vi "Example_RCM.vi"() -> ()   [LabVIEW 2009]
uses:
  RCM.xctl
panel:
  out "Selected?":bool
  in  "Get":bool
  out "Selected Item":string caption="Selected Item:"
  in  "Stop":bool
  in  "Overlay Color":u32(colorbox)=26367 caption="Overlay Color:"
  in  "Frame Color":u32(colorbox)=9868950 caption="Frame Color:"
  in  "Seperator Color":u32(colorbox)=9868950 caption="Separator Color:"
  in  "Font Color":u32(colorbox) caption="Font Color:"
  in  "Font Size":i16=13 caption="Font Size:"
  in  "Font Name":string="Tahoma" caption="Font Name:"
  in  "RCM File Path":path caption="RCM File Path:"
  in  "Control with RCM":bool
  in  "RCM":string(xcontrol)
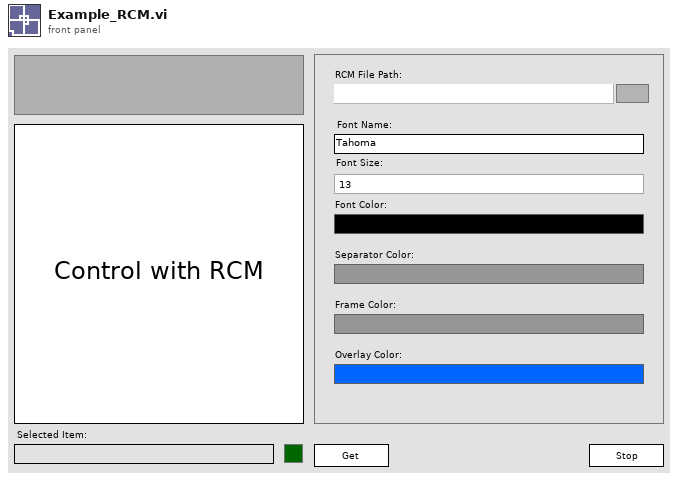
[diagram p1: front panel]
types:
  T1 = typedef "LVPoint32TypeDef.ctl" = cluster{"Horizontal":i32, "Vertical":i32}
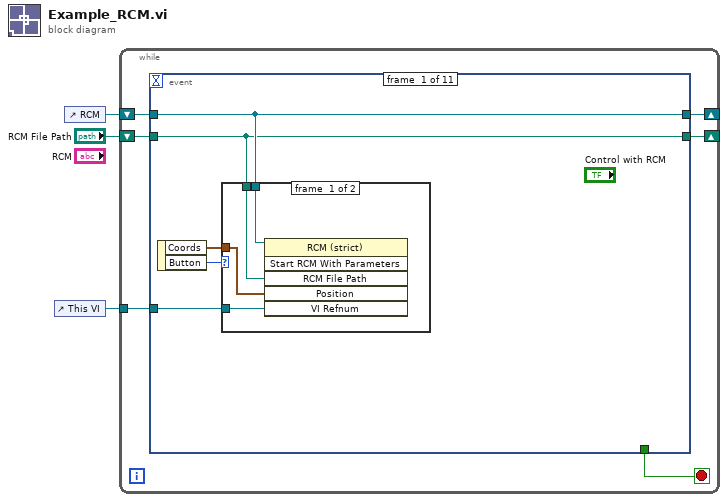
[diagram p0: block diagram]
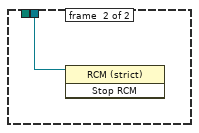
[diagram p2: hidden frame]
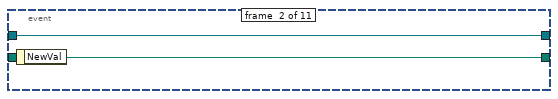
[diagram p3: hidden frame]
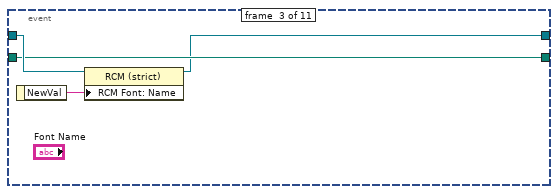
[diagram p4: hidden frame]
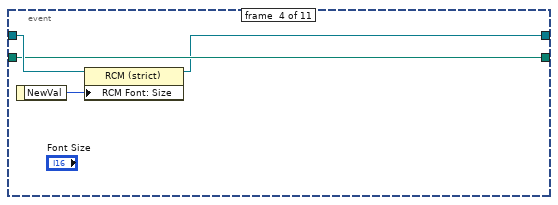
[diagram p5: hidden frame]
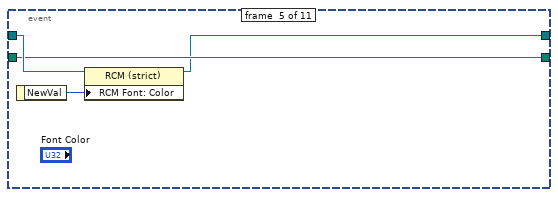
[diagram p6: hidden frame]
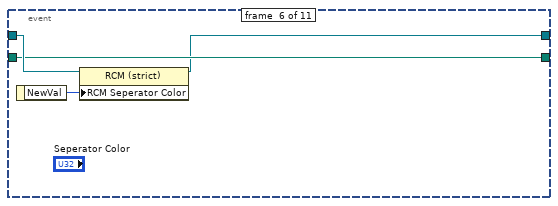
[diagram p7: hidden frame]
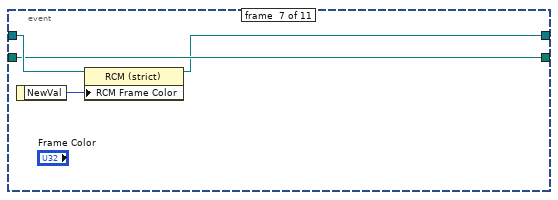
[diagram p8: hidden frame]
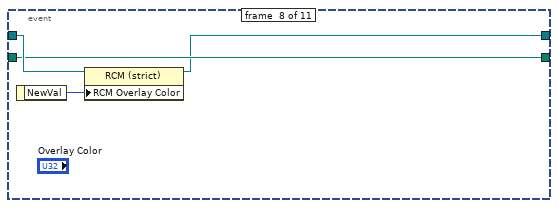
[diagram p9: hidden frame]
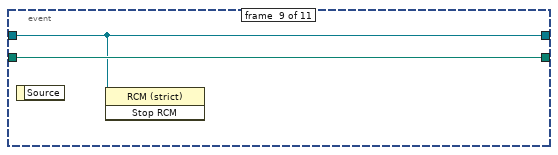
[diagram p10: hidden frame]
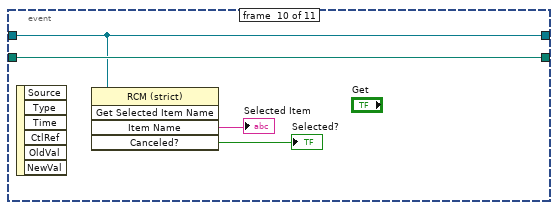
[diagram p11: hidden frame]
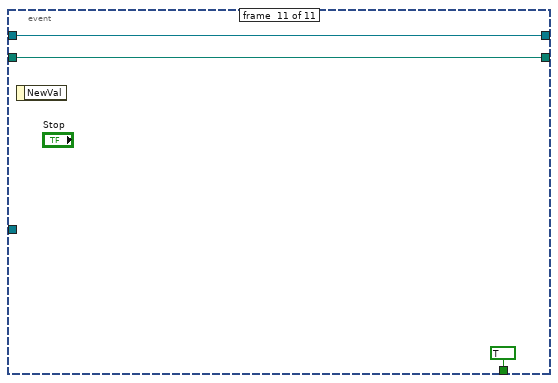
[diagram p12: hidden frame]
diagram:
  n1 = control-ref of="This VI"() -> (w2:refnum<vi>)
  n2 = control-ref of="RCM"() -> (w3:refnum<vi>)
  n3 = while {
    shift-right: [w8] -> _
    shift-left: w3 -> [w9]
    tunnel: w2 -> [w7]
    shift-right: [w5] -> _
    shift-left: "RCM File Path" -> [w6]
    stop <- w4 stop-if-true
    n4 = event shown="[1] \"RCM File Path\": Value Change" {
      selector: _ -> [_ _ _ _ _ _ _ _ _ _ _]
      dyn-events: _ -> [_ _ _ _ _ _ _ _ _ _ _]
      timeout: _ -> [_ _ _ _ _ _ _ _ _ _ _]
      tunnel: w9 -> [w12 w20 w25 w29 w33 w37 w41 w45 w46 w50 w53]
      tunnel: [w12 w20 w23 w27 w31 w35 w39 w43 w46 w50 w53] -> w8
      tunnel: w7 -> [w11 _ _ _ _ _ _ _ _ _ _]
      tunnel: [w10 w21 w24 w28 w32 w36 w40 w44 w47 w51 w54] -> w5
      tunnel: w6 -> [w10 _ w24 w28 w32 w36 w40 w44 w47 w51 w54]
      tunnel: [_ _ _ _ _ _ _ _ _ _ TRUE] -> w4
      event #0 {
        n5 = event-data() -> ("Coords"=w13:T1, "Button"=w14:u16)  [unwired: 1 in]
        n6 = case shown="2" w14 {
          tunnel: w13 -> [w16 _]
          tunnel: w12 -> [w18 w19]
          tunnel: w11 -> [w17 _]
          tunnel: w10 -> [w15 _]
          frame #0 {
            n7 = invoke class="RCM (strict)" method="Start RCM With Parameters"(reference=w18, "RCM File Path"=w15, "Position"=w16, "VI Refnum"=w17) -> ()  [unwired: 2 in, 6 out]
          }
          frame #1 {
            n8 = invoke class="RCM (strict)" method="Stop RCM"(reference=w19) -> ()  [unwired: 2 in, 3 out]
          }
        }
      }
      event #1 {
        n9 = event-data() -> ("NewVal"=w21:path)  [unwired: 1 in]
      }
      event #2 {
        n10 = event-data() -> ("NewVal"=w22:string)  [unwired: 1 in]
        n11 = property class="RCM (strict)"(reference=w25, "RCM Font: Name"=w22) -> (reference out=w23:refnum<vi>)  [unwired: 1 in, 1 out]
      }
      event #3 {
        n12 = event-data() -> ("NewVal"=w26:i16)  [unwired: 1 in]
        n13 = property class="RCM (strict)"(reference=w29, "RCM Font: Size"=w26) -> (reference out=w27:refnum<vi>)  [unwired: 1 in, 1 out]
      }
      event #4 {
        n14 = event-data() -> ("NewVal"=w30:u32)  [unwired: 1 in]
        n15 = property class="RCM (strict)"(reference=w33, "RCM Font: Color"=w30) -> (reference out=w31:refnum<vi>)  [unwired: 1 in, 1 out]
      }
      event #5 {
        n16 = event-data() -> ("NewVal"=w34:u32)  [unwired: 1 in]
        n17 = property class="RCM (strict)"(reference=w37, "RCM Seperator Color"=w34) -> (reference out=w35:refnum<vi>)  [unwired: 1 in, 1 out]
      }
      event #6 {
        n18 = event-data() -> ("NewVal"=w38:u32)  [unwired: 1 in]
        n19 = property class="RCM (strict)"(reference=w41, "RCM Frame Color"=w38) -> (reference out=w39:refnum<vi>)  [unwired: 1 in, 1 out]
      }
      event #7 {
        n20 = event-data() -> ("NewVal"=w42:u32)  [unwired: 1 in]
        n21 = property class="RCM (strict)"(reference=w45, "RCM Overlay Color"=w42) -> (reference out=w43:refnum<vi>)  [unwired: 1 in, 1 out]
      }
      event #8 {
        n22 = event-data() -> ()  [unwired: 1 in, 1 out]
        n23 = invoke class="RCM (strict)" method="Stop RCM"(reference=w46) -> ()  [unwired: 2 in, 3 out]
      }
      event #9 {
        n24 = event-data() -> ()  [unwired: 1 in, 6 out]
        n25 = invoke class="RCM (strict)" method="Get Selected Item Name"(reference=w50) -> ("Item Name"=→"Selected Item":string, "Canceled?"=→"Selected?":bool)  [unwired: 4 in, 3 out]
      }
      event #10 {
        n26 = event-data() -> ()  [unwired: 1 in, 1 out]
      }
    }
  }
